vi "Gripper Control Loop.vi"() -> ()   [LabVIEW 2017]
uses:
  Typedef/Controller Message.ctl
  <vilib>/Rock Robotics/WPI/MotorControl/WPI_MotorControlDeviceRef.ctl
  <vilib>/Rock Robotics/WPI/MotorControl/WPI_MotorControlType.ctl
  <vilib>/Rock Robotics/SystemInterfaces/DIO/FPGA_DIOPWMChannel.ctl
  <vilib>/Rock Robotics/WPI/PWM/WPI_PWMDeadband.ctl
  <vilib>/Rock Robotics/SystemInterfaces/DIO/FPGA_DIOChannel.ctl
  Typedef/FGVAction.ctl
  <vilib>/addons/control/pid/pid.llb/PID (DBL).vi
  SimulatorVIs/Simulation Input Global.vi
  <vilib>/addons/control/pid/NI_PID_pid.lvlib
panel:
  out "Plant Input":dbl(graph)
  in  "output range":cluster{"output high":dbl, "output low":dbl}={"output high"=100.0, "output low"=-1.0} {"output low" format="%.2f"; "output high" format="%.2f"}
  in  "PID gains":T1={"proportional gain (Kc)"=11.9, "integral time (Ti, min)"=0.004, "derivative time (Td, min)"=0.0} {"derivative time (Td, min)" format="%.3f"; "integral time (Ti, min)" format="%.3f"; "proportional gain (Kc)" format="%.3f"}
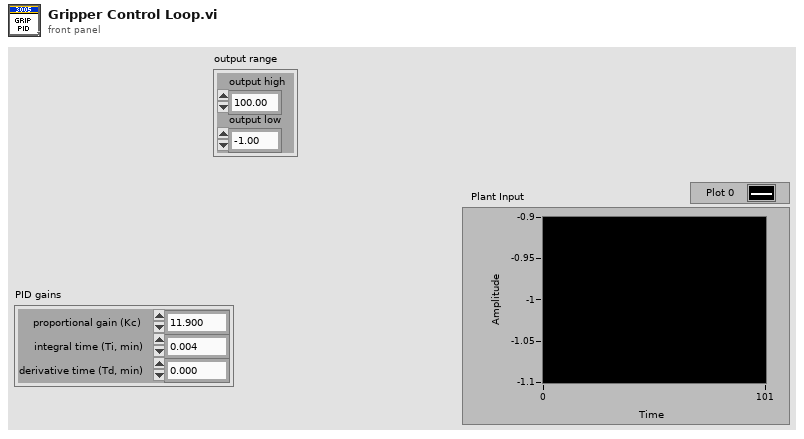
[diagram p1: front panel]
types:
  T1 = cluster{"proportional gain (Kc)":dbl, "integral time (Ti, min)":dbl, "derivative time (Td, min)":dbl}
  T2 = typedef "Controller Message.ctl" = cluster{"Setpoint":dbl, "Manual":bool}
  T3 = typedef "WPI_MotorControlDeviceRef.ctl" = cluster{"DeviceStatus":errorcluster, "Type":T4, "PWM":cluster{"PWM Channel":T5, "DeadBand":T6}, "CAN":cluster{"Device Number":u8, "SetOutput VI Ref":variant, "GetOutput VI Ref":variant, "Enable VI Ref":variant, "Disable VI Ref":variant, "Data":variant}, "Invert":bool, "DIO PWM":cluster{"PWM \"Enable\" Channel":T5, "DIOChannel":T7, "PWM Rate":dbl}}
  T4 = typedef "WPI_MotorControlType.ctl" = enum16{"PWM", "CAN", "DIO PWM"}
  T5 = typedef "FPGA_DIOPWMChannel.ctl" = enum8{"PWM 0", "PWM 1", "PWM 2", "PWM 3", "PWM 4", "PWM 5", "PWM 6", "PWM 7", "PWM 8", "PWM 9", "PWM MXP 0", "PWM MXP 1", "PWM MXP 2", "PWM MXP 3", "PWM MXP 4", "PWM MXP 5", "PWM MXP 6", "PWM MXP 7", "PWM MXP 8", "PWM MXP 9", "Invalid"}
  T6 = typedef "WPI_PWMDeadband.ctl" = cluster{"Name":string, "maxPositivePwm":i32, "minPositivePwm":i32, "centerPwm":i32, "maxNegativePwm":i32, "minNegativePwm":i32, "angularRange":u16}
  T7 = typedef "FPGA_DIOChannel.ctl" = enum8{"DIO 0", "DIO 1", "DIO 2", "DIO 3", "DIO 4", "DIO 5", "DIO 6", "DIO 7", "DIO 8", "DIO 9", "DIO MXP 0", "DIO MXP 1", "DIO MXP 2", "DIO MXP 3", "DIO MXP 4", "DIO MXP 5", "DIO MXP 6", "DIO MXP 7", "DIO MXP 8", "DIO MXP 9", "DIO MXP 10", "DIO MXP 11", "DIO MXP 12", "DIO MXP 13", "DIO MXP 14", "DIO MXP 15", "SPI Port CS1", "SPI Port CS2", "SPI Port CS3", "SPI Port MISO", "SPI Port MOSI", "Invalid"}
  T8 = cluster{"Setpoint":dbl, "notifier out":refnum<notifier>, "Output":dbl, "GripperMotorL":T3, "GripperMotorR":T3}
  T9 = typedef "FGVAction.ctl" = enum16{"get", "set"}
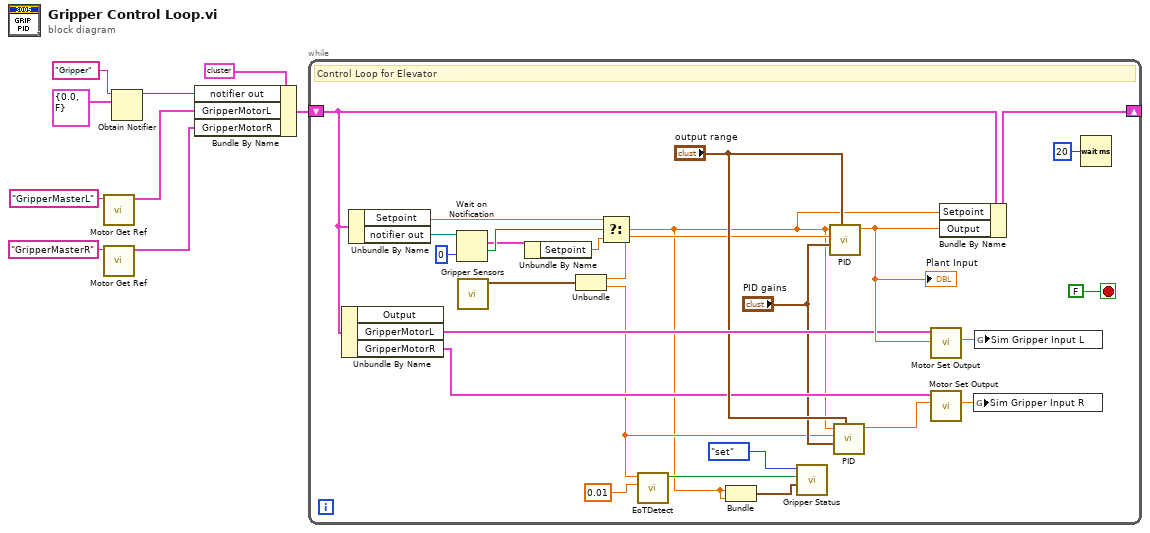
[diagram p0: block diagram]
diagram:
  n1 = call "Motor Get Ref.vi"("refnum name"="GripperMasterL") -> ("MotorControlDevRef"=w5:T3)  [unwired: 10 in]
  n2 = call "Motor Get Ref.vi"("refnum name"="GripperMasterR") -> ("MotorControlDevRef"=w4:T3)  [unwired: 10 in]
  n3 = Obtain Notifier(name (unnamed)="Gripper", notification data type=T2 {"Setpoint"=0.0, "Manual"=FALSE}) -> (notifier out=w7:refnum<notifier>)  [unwired: 2 in, 2 out]
  n4 = Bundle By Name(cluster=T8 {"Setpoint"=0.0, "notifier out"=refnum, "Output"=0.0, "GripperMotorL"={"DeviceStatus"={"status"=FALSE, "code"=0, "source"=""}, "Type"=enum."PWM", "PWM"={"PWM Channel"=enum."Invalid", "DeadBand"={"Name"="", "maxPositivePwm"=0, "minPositivePwm"=0, "centerPwm"=0, "maxNegativePwm"=0, "minNegativePwm"=0, "angularRange"=0}}, "CAN"={"Device Number"=0, "SetOutput VI Ref"=variant(enum8{"Percent VBus", "Current", "Speed", "Position", "Voltage"} enum."Percent VBus"), "GetOutput VI Ref"=variant(refnum<k1> refnum), "Enable VI Ref"=variant(dbl 12.0), "Disable VI Ref"=variant(enum8{"Percent VBus", "Speed", "Position", "Slave", "Unchanged / Invalid"} enum."Percent VBus"), "Data"=variant(enum16{"Controller 1"} enum."Controller 1")}, "Invert"=FALSE, "DIO PWM"={"PWM \"Enable\" Channel"=enum."Invalid", "DIOChannel"=enum."Invalid", "PWM Rate"=0.0}}, "GripperMotorR"={"DeviceStatus"={"status"=FALSE, "code"=0, "source"=""}, "Type"=enum."PWM", "PWM"={"PWM Channel"=enum."Invalid", "DeadBand"={"Name"="", "maxPositivePwm"=0, "minPositivePwm"=0, "centerPwm"=0, "maxNegativePwm"=0, "minNegativePwm"=0, "angularRange"=0}}, "CAN"={"Device Number"=0, "SetOutput VI Ref"=variant(enum8{"Percent VBus", "Current", "Speed", "Position", "Voltage"} enum."Percent VBus"), "GetOutput VI Ref"=variant(refnum<k1> refnum), "Enable VI Ref"=variant(dbl 12.0), "Disable VI Ref"=variant(enum8{"Percent VBus", "Speed", "Position", "Slave", "Unchanged / Invalid"} enum."Percent VBus"), "Data"=variant(enum16{"Controller 1"} enum."Controller 1")}, "Invert"=FALSE, "DIO PWM"={"PWM \"Enable\" Channel"=enum."Invalid", "DIOChannel"=enum."Invalid", "PWM Rate"=0.0}}}, "notifier out"=w7, "GripperMotorL"=w5, "GripperMotorR"=w4) -> (w8:T8)
  n5 = while {
    shift-right: [w31] -> _
    shift-left: w8 -> [w30]
    stop <- FALSE stop-if-true
    # "Control Loop for Elevator"
    n6 = Unbundle By Name(w30) -> ("GripperMotorL"=w26:T3, "GripperMotorR"=w24:T3)  [unwired: 1 out]
    n7 = Unbundle By Name(w30) -> ("Setpoint"=w32:dbl, "notifier out"=w34:refnum<notifier>)
    n8 = Wait on Notification(notifier=w34, timeout in ms (-1)=0) -> (notification=w11:T2, timed out?=w33:bool)  [unwired: 2 in, 2 out]
    n9 = call "Gripper Sensors.vi"() -> ("Gripper Values"=w19:cluster{"Left":dbl, "Right":dbl})  [unwired: 10 in, 1 out]
    n10 = Unbundle By Name(w11) -> ("Setpoint"=w10:dbl)
    n11 = Unbundle(w19) -> ("Left"=w18:dbl, "Right"=w16:dbl)
    n12 = Select(t=w32, s=w33, f=w10) -> (s? t:f=w13:dbl)
    n13 = call "EoTDetect.vi"("Tolerance"=0.01, "Sensor"=w16) -> ("EoT? (F)"=w15:bool)  [unwired: 9 in]
    n14 = Bundle("Setpoint"=w13, "Setpoint"=w13) -> (w12:cluster{"Setpoint":dbl, "Setpoint":dbl})  [unwired: 1 in]
    n15 = call "Gripper Status.vi"("Input"=w12, "Moving? (F)"=w15, "Action"=FGVAction."set") -> ()  [unwired: 6 in, 3 out]
    n16 = call-poly <vilib>:"PID.vi"("output range"="output range", "PID gains"="PID gains", "process variable"=w18, "setpoint"=w13) -> ("output"=w27:dbl)  [unwired: 6 in, 1 out]
    "Plant Input" <- w27
    n17 = call-poly <vilib>:"PID.vi"("output range"="output range", "PID gains"="PID gains", "process variable"=w16, "setpoint"=w13) -> ("output"=w22:dbl)  [unwired: 6 in, 1 out]
    n18 = call "Motor Set Output.vi"("output"=w27, "DriveMotor"=w26) -> ("Motor Output"=w21:dbl)  [unwired: 9 in]
    n19 = call "Motor Set Output.vi"("output"=w22, "DriveMotor"=w24) -> ("Motor Output"=w20:dbl)  [unwired: 9 in]
    n20 = Bundle By Name(cluster=w30, "Setpoint"=w13, "Output"=w27) -> (w31:T8)
    n21 = global write "Simulation Input Global.vi" "Sim Gripper Input R"(w20) -> ()
    n22 = global write "Simulation Input Global.vi" "Sim Gripper Input L"(w21) -> ()
    n23 = Wait (ms)(milliseconds to wait=u32 20) -> ()  [unwired: 1 out]
  }
